vi "AuMT8852B EDR CW Measurement Results.vi"(8 "error in (no error)":errorcluster, 11 "VISA session":refnum<visa-resource-name>) -> (0 "error out":errorcluster, 2 "error code":i32, 3 "VISA session out":refnum<visa-resource-name>, 4 "Results":T1 {"RMS DEVM" format="%.3f"; "Peak DEVM" format="%.3f"; "RMS power (dBm)" format="%.2f"; "Peak power (dBm)" format="%.2f"})   [LabVIEW 2017]
doc: "Anritsu MT8852B Bluetooth Tester\n\nReturns the results of the ECW measurement.\n\nOUTPUTS\nResults - measurements made during the test."
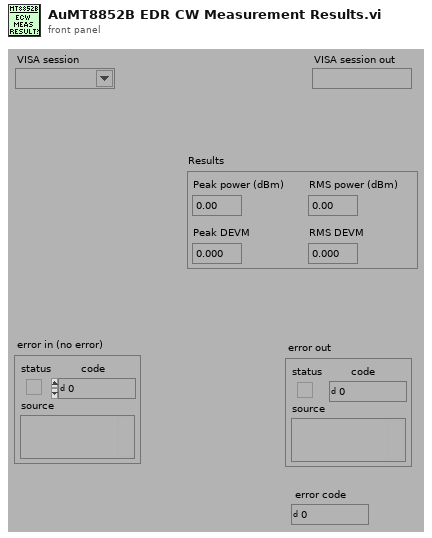
[diagram p1: front panel]
types:
  T1 = cluster{"Peak power (dBm)":dbl, "RMS power (dBm)":dbl, "Peak DEVM":dbl, "RMS DEVM":dbl}
  T2 = enum16{"Simulate", "Range check", "Cache", "Query instrument status"}
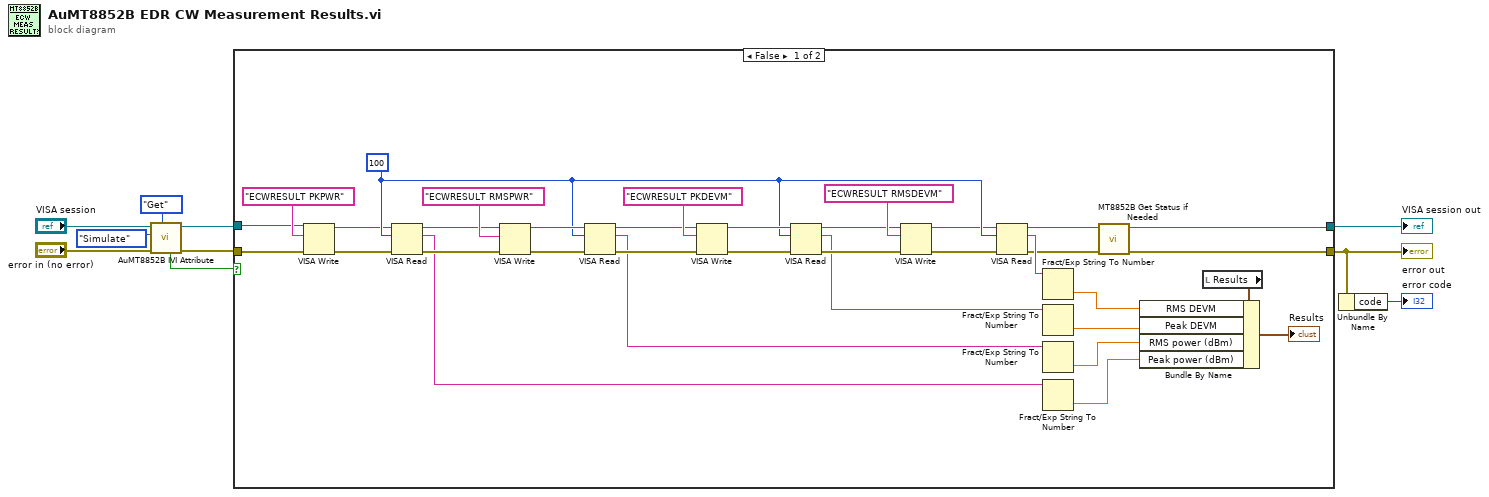
[diagram p0: block diagram]
diagram:
  n1 = call <instrlib>:"AuMT8852B IVI Attribute.vi"("Set/Get (Set)"=enum16{"Set", "Get"}."Get", "error in (no error)"="error in (no error)", "Flag (Simulate)"=T2."Simulate", "VISA session"="VISA session") -> ("error out"=w7:errorcluster, "VISA session out"=w9:refnum<visa-resource-name>, "Value out"=w3:bool)  [unwired: 5 in]
  n2 = case shown="False" w3 {
    tunnel: [w42 w47] -> w10
    tunnel: [w41 w46] -> w1
    tunnel: w9 -> [w44 w47]
    tunnel: w7 -> [w43 w46]
    frame False {
      w26 = u32 100 ("byte count (0)")
      n3 = VISA Write(VISA resource name=w44, write buffer="ECWRESULT PKPWR" ("write buffer (\"\")"), error in (no error)=w43) -> (VISA resource name out=w12:refnum<visa-resource-name>, error out=w13:errorcluster)  [unwired: 1 out]
      n4 = VISA Read(VISA resource name=w12, byte count=w26, error in (no error)=w13) -> (VISA resource name out=w11:refnum<visa-resource-name>, read buffer=w20:string, error out=w38:errorcluster)  [unwired: 1 out]
      n5 = VISA Write(VISA resource name=w11, write buffer="ECWRESULT RMSPWR" ("write buffer (\"\")"), error in (no error)=w38) -> (VISA resource name out=w40:refnum<visa-resource-name>, error out=w37:errorcluster)  [unwired: 1 out]
      n6 = VISA Read(VISA resource name=w40, byte count=w26, error in (no error)=w37) -> (VISA resource name out=w32:refnum<visa-resource-name>, read buffer=w31:string, error out=w33:errorcluster)  [unwired: 1 out]
      n7 = VISA Write(VISA resource name=w32, write buffer="ECWRESULT PKDEVM" ("write buffer (\"\")"), error in (no error)=w33) -> (VISA resource name out=w34:refnum<visa-resource-name>, error out=w36:errorcluster)  [unwired: 1 out]
      n8 = VISA Read(VISA resource name=w34, byte count=w26, error in (no error)=w36) -> (VISA resource name out=w28:refnum<visa-resource-name>, read buffer=w27:string, error out=w29:errorcluster)  [unwired: 1 out]
      n9 = VISA Write(VISA resource name=w28, write buffer="ECWRESULT RMSDEVM" ("write buffer (\"\")"), error in (no error)=w29) -> (VISA resource name out=w22:refnum<visa-resource-name>, error out=w24:errorcluster)  [unwired: 1 out]
      n10 = VISA Read(VISA resource name=w22, byte count=w26, error in (no error)=w24) -> (VISA resource name out=w21:refnum<visa-resource-name>, read buffer=w25:string, error out=w23:errorcluster)  [unwired: 1 out]
      n11 = Fract/Exp String To Number(string=w25) -> (number=w19:dbl)  [unwired: 3 in, 1 out]
      n12 = Fract/Exp String To Number(string=w27) -> (number=w18:dbl)  [unwired: 3 in, 1 out]
      n13 = Fract/Exp String To Number(string=w31) -> (number=w17:dbl)  [unwired: 3 in, 1 out]
      n14 = Fract/Exp String To Number(string=w20) -> (number=w16:dbl)  [unwired: 3 in, 1 out]
      n15 = call <instrlib>:"MT8852B Get Status if Needed.vi"("error in (no error)"=w23, "VISA session"=w21) -> ("error out"=w41:errorcluster, "VISA session out"=w42:refnum<visa-resource-name>)  [unwired: 8 in]
      n16 = local read "Results"() -> (w15:T1)
      n17 = Bundle By Name(cluster=w15, "RMS DEVM"=w19, "Peak DEVM"=w18, "RMS power (dBm)"=w17, "Peak power (dBm)"=w16) -> (→"Results":T1)
    }
    frame True {
    }
  }
  "error out" <- w1
  "VISA session out" <- w10
  n18 = Unbundle By Name(w1) -> ("code"=→"error code":i32)
